vi "webdsocket.vi"() -> ()   [LabVIEW 2013]
uses:
  <vilib>/MediaMongrels Ltd/WebSockets/WebSockets/WebSockets.lvlib
panel:
  in  "Name":string
  out "Data":string
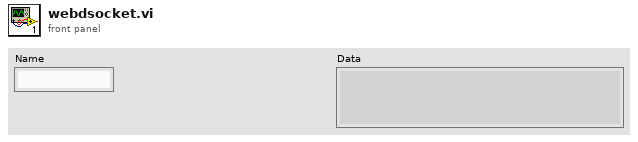
[diagram p1: front panel]
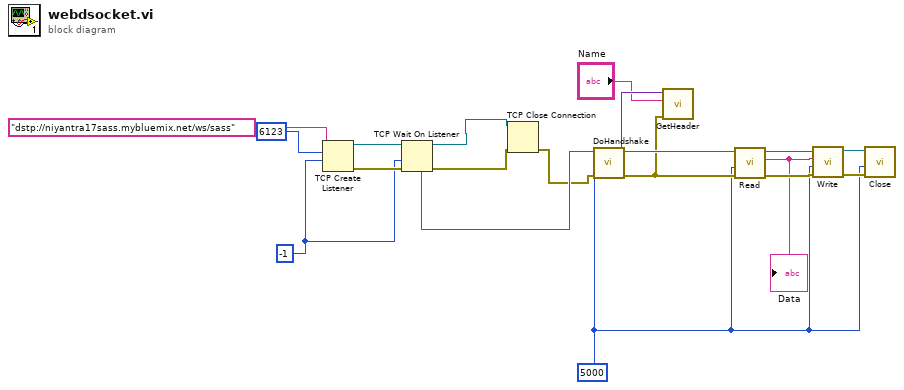
[diagram p0: block diagram]
diagram:
  w4 = 5000 ("timeout ms (5000)")
  w5 = -1 ("timeout ms (25000)")
  n1 = TCP Create Listener(9:w5, 10:u16 6123 ("port"), 11:"dstp://niyantra17sass.mybluemix.net/ws/sass" ("service name")) -> (0:w6:errorcluster, 3:w7:refnum<k5>)  [unwired: 2 in, 1 out]
  n2 = TCP Wait On Listener(8:w6, 9:w5, 11:w7) -> (0:w11:errorcluster, 3:w10:refnum<k5>, 4:w9:refnum<k5>)  [unwired: 1 in, 2 out]
  n3 = TCP Close Connection(connection ID=w10, error in (no error)=w11) -> (error out=w3:errorcluster)  [unwired: 1 in, 1 out]
  n4 = call <vilib>:"DoHandshake.vi"("error in (no error)"=w3, "timeout ms (5000)"=w4, "WebSocket Connection in"=w9) -> ("error out"=w13:errorcluster, "Headers Out"=w14:variant, "WebSocket Connection out"=w15:refnum<k5>)  [unwired: 5 in, 1 out]
  n5 = call <vilib>:"GetHeader.vi"("error in (no error)"=w13, "Name"="Name", "Headers In"=w14) -> ()  [unwired: 5 in, 4 out]
  n6 = call <vilib>:"Read.vi"("error in (no error)"=w13, "timeout ms (5000)"=w4, "WebSocket Connection in"=w15) -> ("error out"=w16:errorcluster, "Data"=w12:string, "WebSocket Connection out"=w17:refnum<k5>)  [unwired: 5 in, 1 out]
  "Data" <- w12
  n7 = call <vilib>:"Write.vi"("error in (no error)"=w16, "timeout ms (5000)"=w4, "Data"=w12, "WebSocket Connection in"=w17) -> ("error out"=w19:errorcluster, "WebSocket Connection out"=w18:refnum<k5>)  [unwired: 6 in]
  n8 = call <vilib>:"Close.vi"("error in (no error)"=w19, "timeout ms (5000)"=w4, "WebSocket Connection in"=w18) -> ()  [unwired: 7 in, 2 out]
